vi "IMAQ Read Image File(Float32 Ex).vi"(7 "File Path":path, 8 "error in (no error)":errorcluster, 11 "Image":T1) -> (0 "error out":errorcluster, 3 "Image (duplicate)":T1)   [LabVIEW 2020]
uses:
  <vilib>/vision/Image Controls.llb/IMAQ Image.ctl
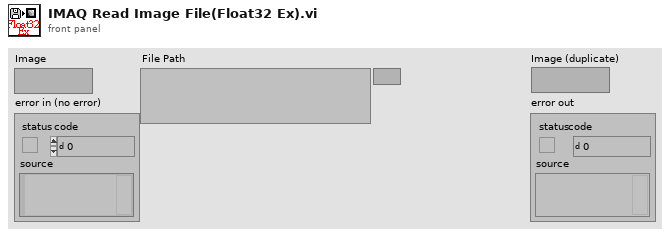
[diagram p1: front panel]
types:
  T1 = typedef "IMAQ Image.ctl" = refnum<image>
  T2 = typedef "Image Type" = u32
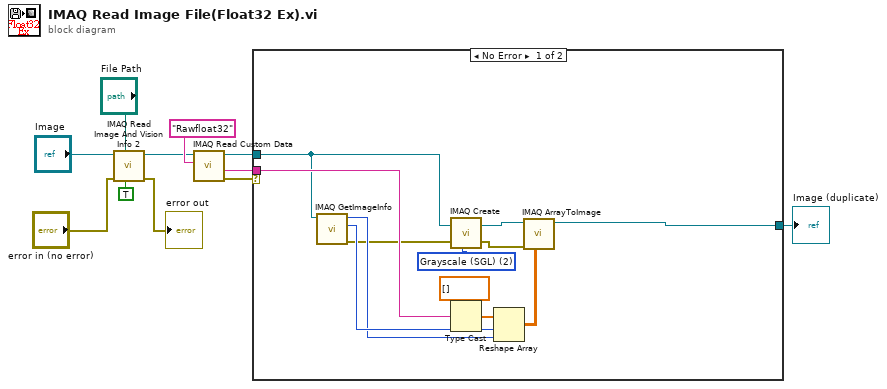
[diagram p0: block diagram]
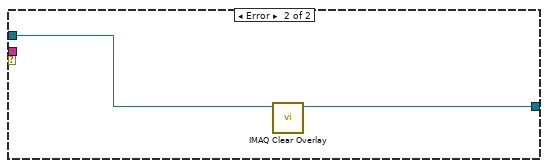
[diagram p2: hidden frame]
diagram:
  n1 = call "IMAQ Read Image And Vision Info 2"("Use File Path Image Type"=TRUE, "File Path"="File Path", "error in (no error)"="error in (no error)", "Image"="Image") -> ("error out"=→"error out":errorcluster, "Image Out"=w9:T1)  [unwired: 5 in, 1 out]
  n2 = call "IMAQ Read Custom Data"("Key"="Rawfloat32", "Image"=w9) -> ("error out"=w2:errorcluster, "Custom Data Out"=w10:string, "Image (duplicate)"=w8:T1)  [unwired: 7 in]
  n3 = case shown="No Error" w2 {
    tunnel: w10 -> [w23 _]
    tunnel: [w14 w24] -> w3
    tunnel: w8 -> [w15 w25]
    frame No Error {
      w20 = T2 2 items=["Grayscale (U8)", "Grayscale (I16)", "Grayscale (SGL)", "Complex (CSG)", "RGB (U32)", "HSL (U32)", "RGB (U64)", "Grayscale (U16)"] ("Image Type")
      n4 = call "IMAQ GetImageInfo"("Image"=w15) -> ("error out"=w13:errorcluster, "Y Resolution"=w18:i32, "X Resolution"=w17:i32)  [unwired: 3 in, 5 out]
      n5 = call "IMAQ Create"("Image Name"=w15, "Image Type"=w20, "error in (no error)"=w13) -> ("New Image"=w19:T1, "error out"=w12:errorcluster)  [unwired: 2 in]
      n6 = Type Cast(type=sgl[] [], x=w23) -> (*(type *) &x=w22:sgl[])
      n7 = Reshape Array(w22, w18, w17) -> (w21:sgl[][])
      n8 = call "IMAQ ArrayToImage"("Image Pixels (Float)"=w21, "error in (no error)"=w12, "Image"=w19) -> ("Image Out"=w14:T1)  [unwired: 7 in, 1 out]
    }
    frame Error {
      n9 = call "IMAQ Clear Overlay"("Image"=w25) -> ("Image Out"=w24:T1)  [unwired: 9 in, 1 out]
    }
  }
  "Image (duplicate)" <- w3
